vi "Initiate Syringe Run.vi"(8 "error in (no error)":errorcluster) -> (0 "error out":errorcluster)   [LabVIEW 2015, in "cRIO-Carbondioxide.lvlib" / "cRIO-CO2.lvlib" / "cRIO-CO2.lvclass"]
uses:
  cRIO-CO2.lvclass
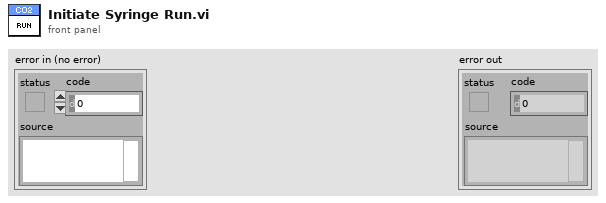
[diagram p1: front panel]
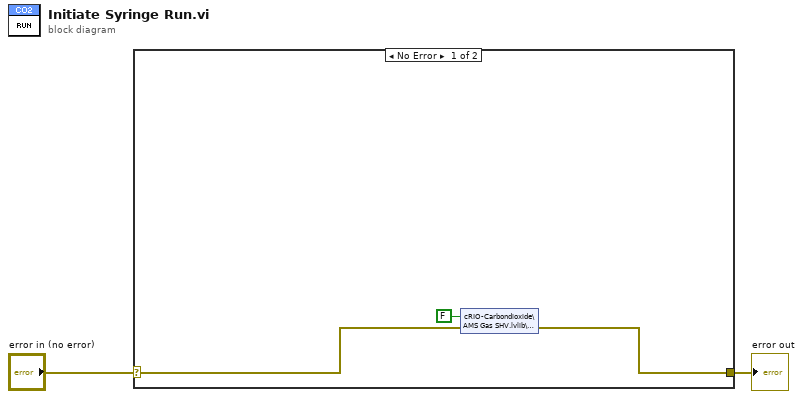
[diagram p0: block diagram]
diagram:
  n1 = case shown="No Error" "error in (no error)" {
    selector: "error in (no error)" -> [w5 w6]
    tunnel: [w4 w6] -> w1
    frame No Error {
      n2 = shared-variable "cRIO-Carbondioxide\\AMS Gas SHV.lvlib\\Cylinder.lvlib\\Home"(FALSE ("Home"), error in=w5) -> (error out=w4:errorcluster)
    }
    frame Error {
    }
  }
  "error out" <- w1
